vi "ROI entry-Init current ROI tool.vi"(8 "error in (no error)":errorcluster) -> (0 "error out":errorcluster)   [LabVIEW 2020]
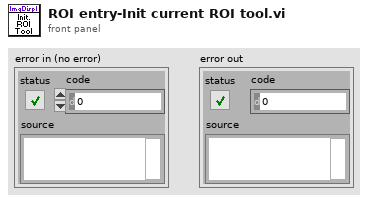
[diagram p1: front panel]
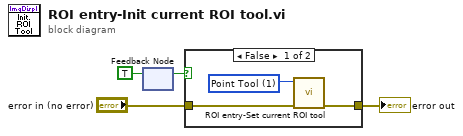
[diagram p0: block diagram]
diagram:
  n1 = feedback #1() -> (w2:bool)  [unwired: 1 in]
  n2 = feedback-in #1(TRUE) -> ()
  n3 = case shown="False" w2 {
    tunnel: [w6 w8] -> w4
    tunnel: "error in (no error)" -> [w5 w8]
    frame False {
      w7 = u32 1 items=["Zoom Tool"=8, "Selection Tool"=0, "Pan Tool"=9, "Point Tool"=1, "Line Tool"=2, "Rectangle Tool"=3, "Rotated Rectangle Tool"=12, "Polyline Tool"=10, "Polygon Tool"=5, "Freehand Tool"=11, "Closed Freehand Tool"=6, "Ellipse Tool"=4, "Annulus Tool"=7] ("Current ROI Tool")
      n4 = call "ROI entry-Set current ROI tool.vi"("error in (no error)"=w5, "Current ROI Tool"=w7) -> ("error out"=w6:errorcluster)  [unwired: 9 in]
    }
    frame True {
    }
  }
  "error out" <- w4
